vi "Write log.vi"(8 "error in (no error)":errorcluster, 10 "Session Handle":T1, 11 "Instr Actor in":refnum<class "Instr Actor.lvclass">) -> (0 "error out":errorcluster, 3 "Instr Actor out":refnum<class "Instr Actor.lvclass">)   [LabVIEW 2014, in "Instrument Library.lvlib" / "Instr Actor.lvclass"]
uses:
  Instr Actor.lvclass
  <userlib>/_Session Fwk/Typedefs/Session Handle.ctl
  <userlib>/_Session Fwk/Session - Root.lvclass
  Instr Actor.lvclass/Instr Actor.ctl
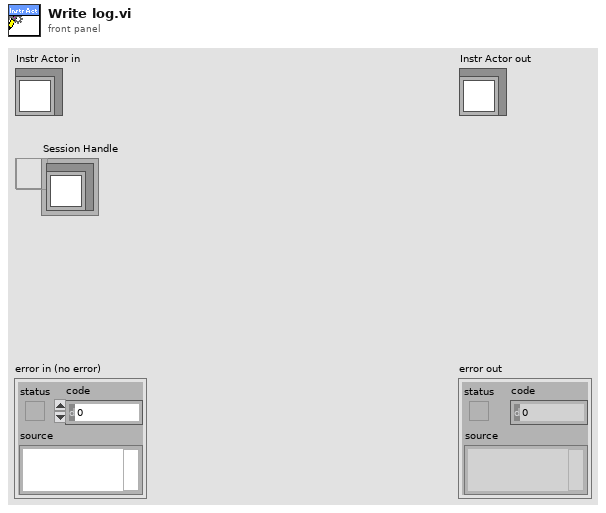
[diagram p1: front panel]
types:
  T1 = typedef "Session - Root.lvclass/Session Handle.ctl" = refnum<data-value>
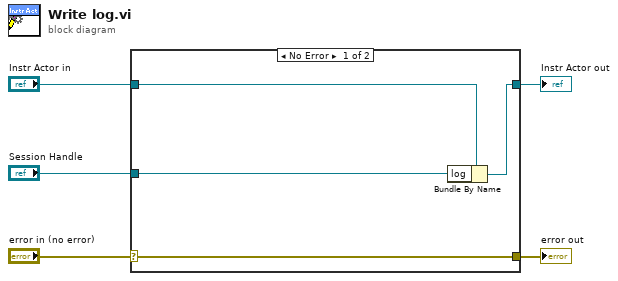
[diagram p0: block diagram]
diagram:
  n1 = case shown="No Error" "error in (no error)" {
    selector: "error in (no error)" -> [w9 w10]
    tunnel: [w9 w10] -> w4
    tunnel: [w7 w11] -> w2
    tunnel: "Instr Actor in" -> [w8 w11]
    tunnel: "Session Handle" -> [w6 _]
    frame No Error {
      n2 = Bundle By Name(cluster=w8, "log"=w6) -> (w7:refnum<class "Instr Actor.lvclass">)
    }
    frame Error {
    }
  }
  "error out" <- w4
  "Instr Actor out" <- w2
